vi "TEST Make Panel Draggable.vi"() -> ()   [LabVIEW 2011]
panel:
  out "current time":timestamp format="%<%I:%M:%S %p\n%x>T"
  in  "stop":bool
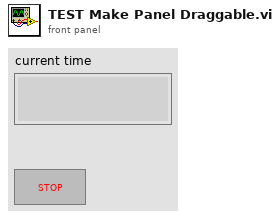
[diagram p1: front panel]
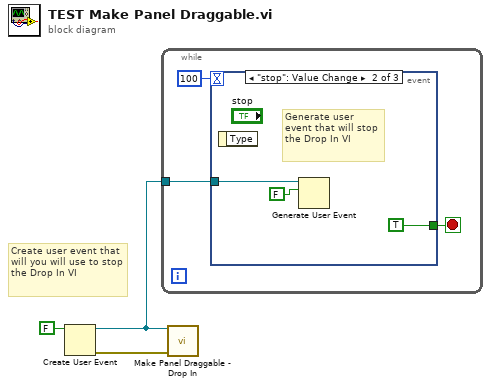
[diagram p0: block diagram]
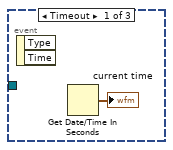
[diagram p2: hidden frame]
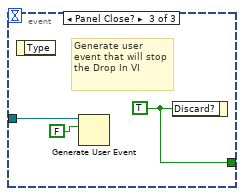
[diagram p3: hidden frame]
diagram:
  # "Create user event that will you will use to stop the Drop In VI"
  n1 = Create User Event(user event datatype=FALSE ("event data")) -> (user event=w2:refnum<user-event>, error out=w1:errorcluster)  [unwired: 1 in]
  n2 = while {
    tunnel: w2 -> [w6]
    stop <- w5 stop-if-true
    n3 = event shown="[1] \"stop\": Value Change" {
      selector: _ -> [_ _ _]
      dyn-events: _ -> [_ _ _]
      timeout: 100 -> [_ _ _]
      tunnel: w6 -> [_ w10 w11]
      tunnel: [_ TRUE w13] -> w5
      event Timeout {
        n4 = event-data() -> ()  [unwired: 1 in, 2 out]
        n5 = Get Date/Time In Seconds() -> (seconds since 1Jan1904=→"current time":timestamp)
      }
      event "stop": Value Change {
        # "Generate user event that will stop the Drop In VI"
        n6 = event-data() -> ()  [unwired: 1 in, 1 out]
        n7 = Generate User Event(user event=w10, event data cluster=FALSE ("event data")) -> ()  [unwired: 1 in, 2 out]
      }
      event Panel Close? {
        w13 = TRUE ("Discard?")
        # "Generate user event that will stop the Drop In VI"
        n8 = event-data() -> ()  [unwired: 1 in, 1 out]
        n9 = Generate User Event(user event=w11, event data cluster=FALSE ("event data")) -> ()  [unwired: 1 in, 2 out]
        n10 = event-data("Discard?"=w13) -> ()  [unwired: 1 in, 1 out]
      }
    }
  }
  n11 = call "Make Panel Draggable - Drop In.vi"("User Event"=w2, "error in (no error)"=w1) -> ()  [unwired: 13 in, 1 out]
